vi "Wave2D_Init Data_BC_Corner.vi"(9 "End Y":cluster{"type":T1, "Value":dbl[][]} {"type" items=["Dirichlet", "Neumann"]}, 10 "Start Y":cluster{"type":T1, "Value":dbl[][]} {"type" items=["Dirichlet", "Neumann"]}, 11 "X":cluster{"type":T1, "Value":dbl[][]} {"type" items=["Dirichlet", "Neumann"]}) -> (2 "X & End Y":dbl[](array[numeric]), 3 "X & Start Y":dbl[](array[numeric]))   [LabVIEW 2017, in "NI_PDE.lvlib"]
uses:
  <vilib>/gmath/NI_PDE.lvlib
  <vilib>/gmath/pde.llb/Common/PDE_BC Type.ctl
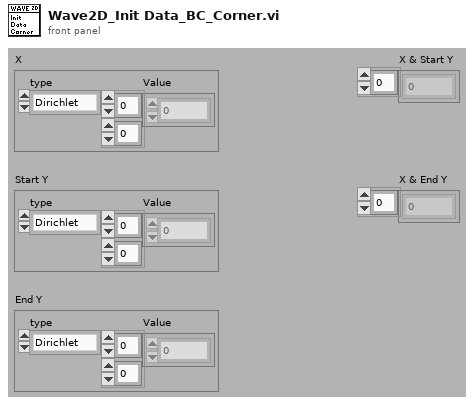
[diagram p1: front panel]
types:
  T1 = typedef "NI_PDE.lvlib/PDE_BC Type.ctl" = i32
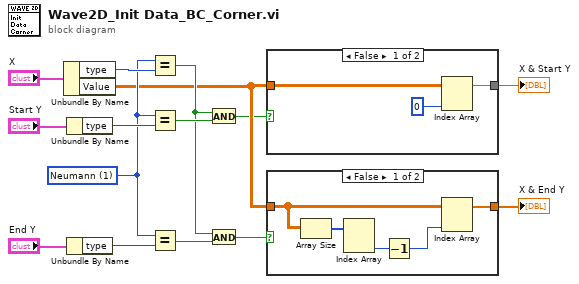
[diagram p0: block diagram]
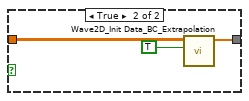
[diagram p2: hidden frame]
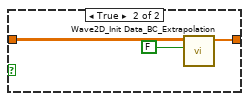
[diagram p3: hidden frame]
diagram:
  w6 = T1 1 items=["Dirichlet", "Neumann"] ("x")
  n1 = Unbundle By Name("X") -> ("type"=w10:T1, "Value"=w3:dbl[][])
  n2 = Unbundle By Name("Start Y") -> ("type"=w13:T1)
  n3 = Unbundle By Name("End Y") -> ("type"=w11:T1)
  n4 = Equal?(x=w6, y=w10) -> (x = y?=w8:bool)
  n5 = Equal?(x=w6, y=w13) -> (x = y?=w9:bool)
  n6 = Equal?(x=w6, y=w11) -> (x = y?=w7:bool)
  n7 = And(x=w8, y=w9) -> (x .and. y?=w2:bool)
  n8 = And(x=w8, y=w7) -> (x .and. y?=w5:bool)
  n9 = case shown="False" w2 {
    tunnel: w3 -> [w17 w21]
    tunnel: [w18 w19] -> w1
    frame False {
      n10 = Index Array(array=w17, index (col)=0 ("disabled index (col)")) -> (element=w18:dbl[])  [unwired: 1 in]
    }
    frame True {
      n11 = call <vilib>:"Wave2D_Init Data_BC_Extrapolation.vi"("start?"=TRUE, "Value"=w21) -> ("Extrapolated Value"=w19:dbl[])  [unwired: 9 out]
    }
  }
  "X & Start Y" <- w1
  n12 = case shown="False" w5 {
    tunnel: w3 -> [w25 w29]
    tunnel: [w26 w27] -> w4
    frame False {
      n13 = Array Size(array=w25) -> (size(s)=w24:i32[])
      n14 = Index Array(array=w24) -> (element #2=w23:i32)  [unwired: 2 in, 1 out]
      n15 = Decrement(x=w23) -> (x-1=w22:i32)
      n16 = Index Array(array=w25, index (col)=w22) -> (element=w26:dbl[])  [unwired: 1 in]
    }
    frame True {
      n17 = call <vilib>:"Wave2D_Init Data_BC_Extrapolation.vi"("start?"=FALSE, "Value"=w29) -> ("Extrapolated Value"=w27:dbl[])  [unwired: 9 out]
    }
  }
  "X & End Y" <- w4
